vi "SEA-9811_ReceiverAndTransmitter_FPGA_9220_IO_simulated_NO_NIVS.vi"() -> ()   [LabVIEW 2015]
doc: "This example demonstrates the receiver's functionality. ARINC data can be received with up to 8 channels which can be configured regarding high- or low-speed data rate, label recognition, parity check, decoder functions or label bit order (CONFIG). Up to sixteen 8-bit labels can be stored for label recognition. Duplicate values if you need fewer labels. For more details, look at the RT frontend example.\n\nCopyright (c) 2013 S.E.A. Datentechnik GmbH, Germany"
uses:
  <vilib>/Platform/TimedLoop/XDataNode/timing_clust.ctl
  <vilib>/Platform/TimedLoop/XDataNode/nitl_modes.ctl
  <vilib>/Platform/TimedLoop/XDataNode/wakeup.ctl
  <vilib>/rvi/Emulation/niFpgaGetClockAttributes.vi
  <vilib>/rvi/Emulation/niFpgaSctlEmulationGetInTimedLoop.vi
  <vilib>/rvi/Emulation/niFpgaEmulationReportErrorSimple.vi
  <vilib>/rvi/Emulation/niFpgaCriticalErrorInLSC.vi
  <vilib>/rvi/Emulation/niFpgaProcessEmulError.vi
  GlobalVar.vi
  <vilib>/rvi/interface/RandomDataEmulation/niFpgaRandomDataHandleErrors.vi
  <vilib>/Platform/TimedLoop/XDataNode/XDataNode.xnode
  <vilib>/rvi/DataTransferAndStorage/Container/XNode/niFpgaContainer.xnode
  <vilib>/rvi/interface/RandomDataEmulation/nirviRandomDataFpgaReadWriteTemplate.vi
  <vilib>/rvi/eio/common/nirviEmuTemplateMethod_errors.vi
  <vilib>/eio/EIOPropertyNode/EIOPropertyNode.xnode
  <vilib>/eio/EIOMethodNode/EIOMethodNode.xnode
  <vilib>/eio/EIONode/EIONode.xnode
  <vilib>/rvi/eio/common/nirviEmuTemplatePropertyGet_errors.vi
  <vilib>/rvi/eio/common/nirviEmuTemplatePropertyGet_noerrors.vi
  <vilib>/rvi/eio/common/nirviEmuTemplatePropertySet_errors.vi
  <vilib>/rvi/eio/common/nirviEmuTemplatePropertySet_noerrors.vi
  <userlib>/FPGA Timekeeper 1.1b0/FPGA Timekeeper.lvlib
  <vilib>/Platform/TimedLoop/XDataNode/XDNodeRunTimeDep.lvlib
panel:
  in  "Rx Label Filter":u8[](array[numeric])=[0, 0, 0, 0, 0, 0, 0, 0, 0, 0, 0, 0, 0, 0, 0, 0]
  in  "RxSimRate(mSec)":u32=5 caption="Count(mSec)"
  out "Pulse":bool
  out "Counter":u32
  in  "AI0_threshold (V)":fxp<+/-,24,5>=5.0
  in  "Pulse length (ms)":u32
  in  "FPGA Loop rate (usec)":u16
  out "9220_AIs":fxp<+/-,24,5>[](array[numeric])
  out "Rx rate us":u32
  out "Elements in FIFO":u32
  out "FPGA Timekeeper time (ns)":u64
  out "FPGA Timekeeper locked":bool
  out "offset from RT time (ns)":i32
  in  "RT time (ns)":u64
  in  "Finished config":bool
  in  "Configure\nchannel":bool
  out "Rx Status":u16 format="%016b"
  out "Tx Status":u8 format="%08b"
  in  "Tx Data":u32=305419896 format="%08x"
  in  "Tx Config Data (TCR)":u16=8192 format="%04x"
  in  "Transmit Data":bool
  out "DMA Overflow":bool
  in  "Rx Channel Number":u8 max=7 step=1
  in  "Rx Config Data (RCR)":u16=32 format="%04x"
  # "Please refer to VI description for instructions!"
  # "Receiver Configuration"
  # "DMA Status"
  # "Transmitter"
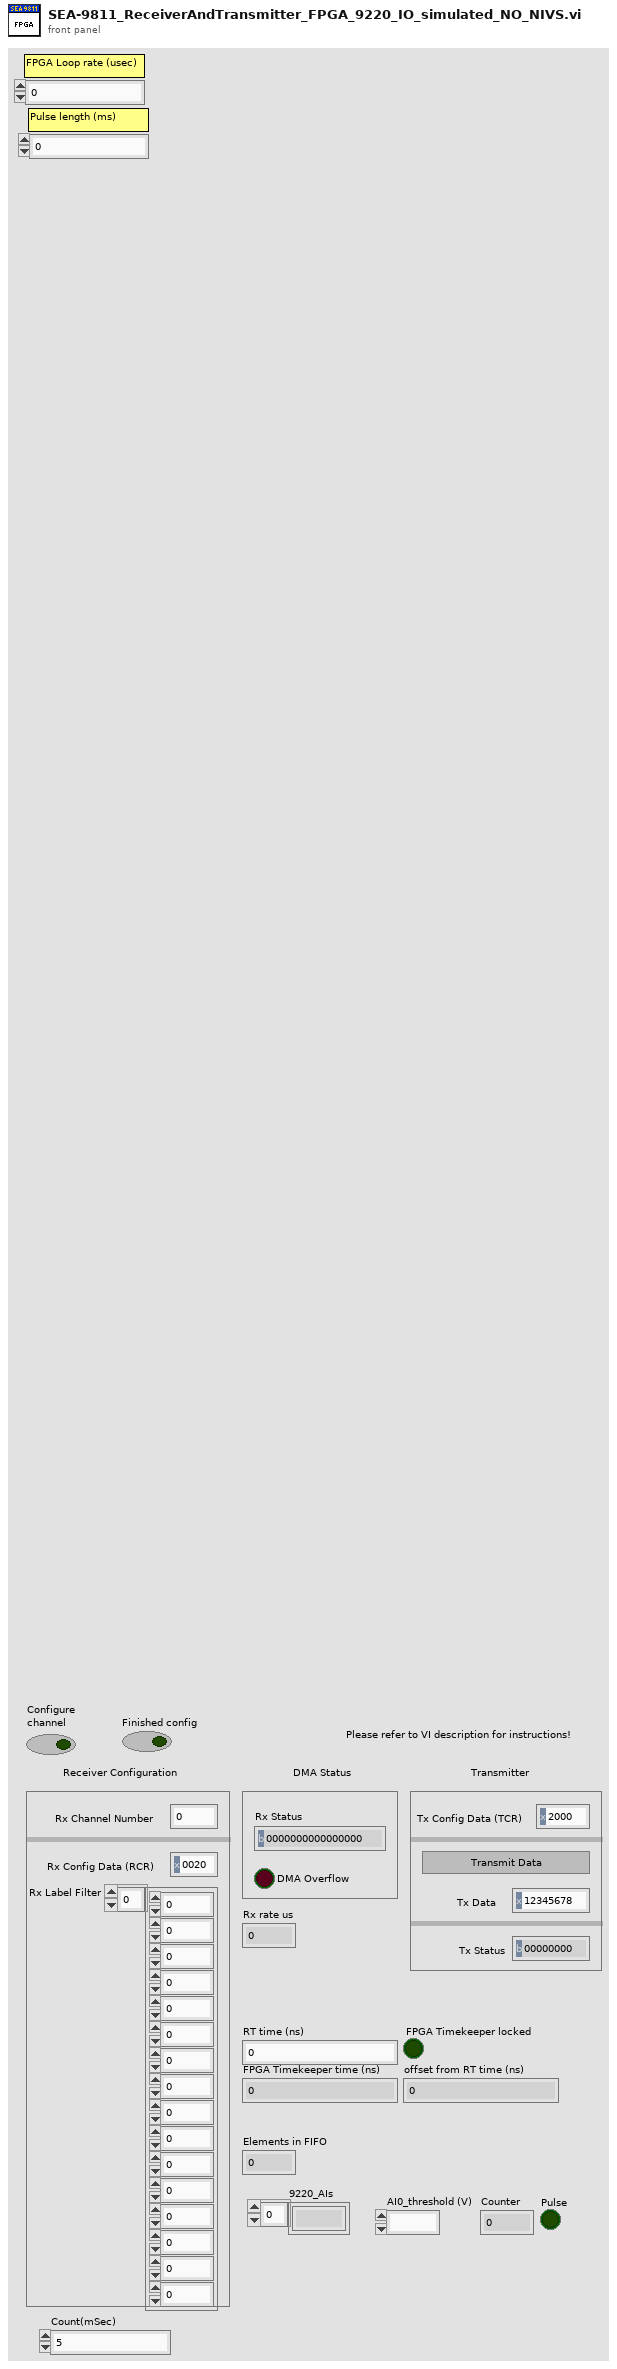
[diagram p1: front panel]
types:
  T1 = cluster{"Rx Label Filter[0]":u8, "Rx Label Filter[1]":u8, "Rx Label Filter[2]":u8, "Rx Label Filter[3]":u8, "Rx Label Filter[4]":u8, "Rx Label Filter[5]":u8, "Rx Label Filter[6]":u8, "Rx Label Filter[7]":u8, "Rx Label Filter[8]":u8, "Rx Label Filter[9]":u8, "Rx Label Filter[10]":u8, "Rx Label Filter[11]":u8, "Rx Label Filter[12]":u8, "Rx Label Filter[13]":u8, "Rx Label Filter[14]":u8, "Rx Label Filter[15]":u8}
  T2 = typedef "XDNodeRunTimeDep.lvlib/timing_clust.ctl" = cluster{"Expected End [f-1]":u64, "Actual End [f-1]":u64, "Finished Late? [f-1]":bool, "Expected End [i-1]":u64, "Actual End [i-1]":u64, "Finished Late? [i-1]":bool, "Expected Start [i]":u64, "Actual Start [i]":u64, "Expected Start [f]":u64, "Actual Start [f]":u64, "Source Name":string, "Structure Name":string, "Period":i64, "Deadline":i64, "Offset":i64, "Start":i64, "Priority":i32, "Timeout":i32, "Mode":T3, "Wakeup Reason":T4, "Error":errorcluster, "Source Type":string, "Secondary Source Type":string, "Global End Time":u64, "Global Start Time":u64, "Frame Duration":u64, "Iteration Duration":u64, "Assigned CPU":i32, "I/O Scan Engine Mode":u32}
  T3 = typedef "XDNodeRunTimeDep.lvlib/nitl_modes.ctl" = enum32{"No Change", "Process missed periods, maintain original phase", "Discard missed periods, maintain original phase", "Process missed periods, ignore original phase", "Discard missed periods, ignore original phase"}
  T4 = typedef "XDNodeRunTimeDep.lvlib/wakeup.ctl" = enum32{"Normal", "Aborted", "Asynchronous wakeup", "Timing source error", "Timed loop error", "Timeout"}
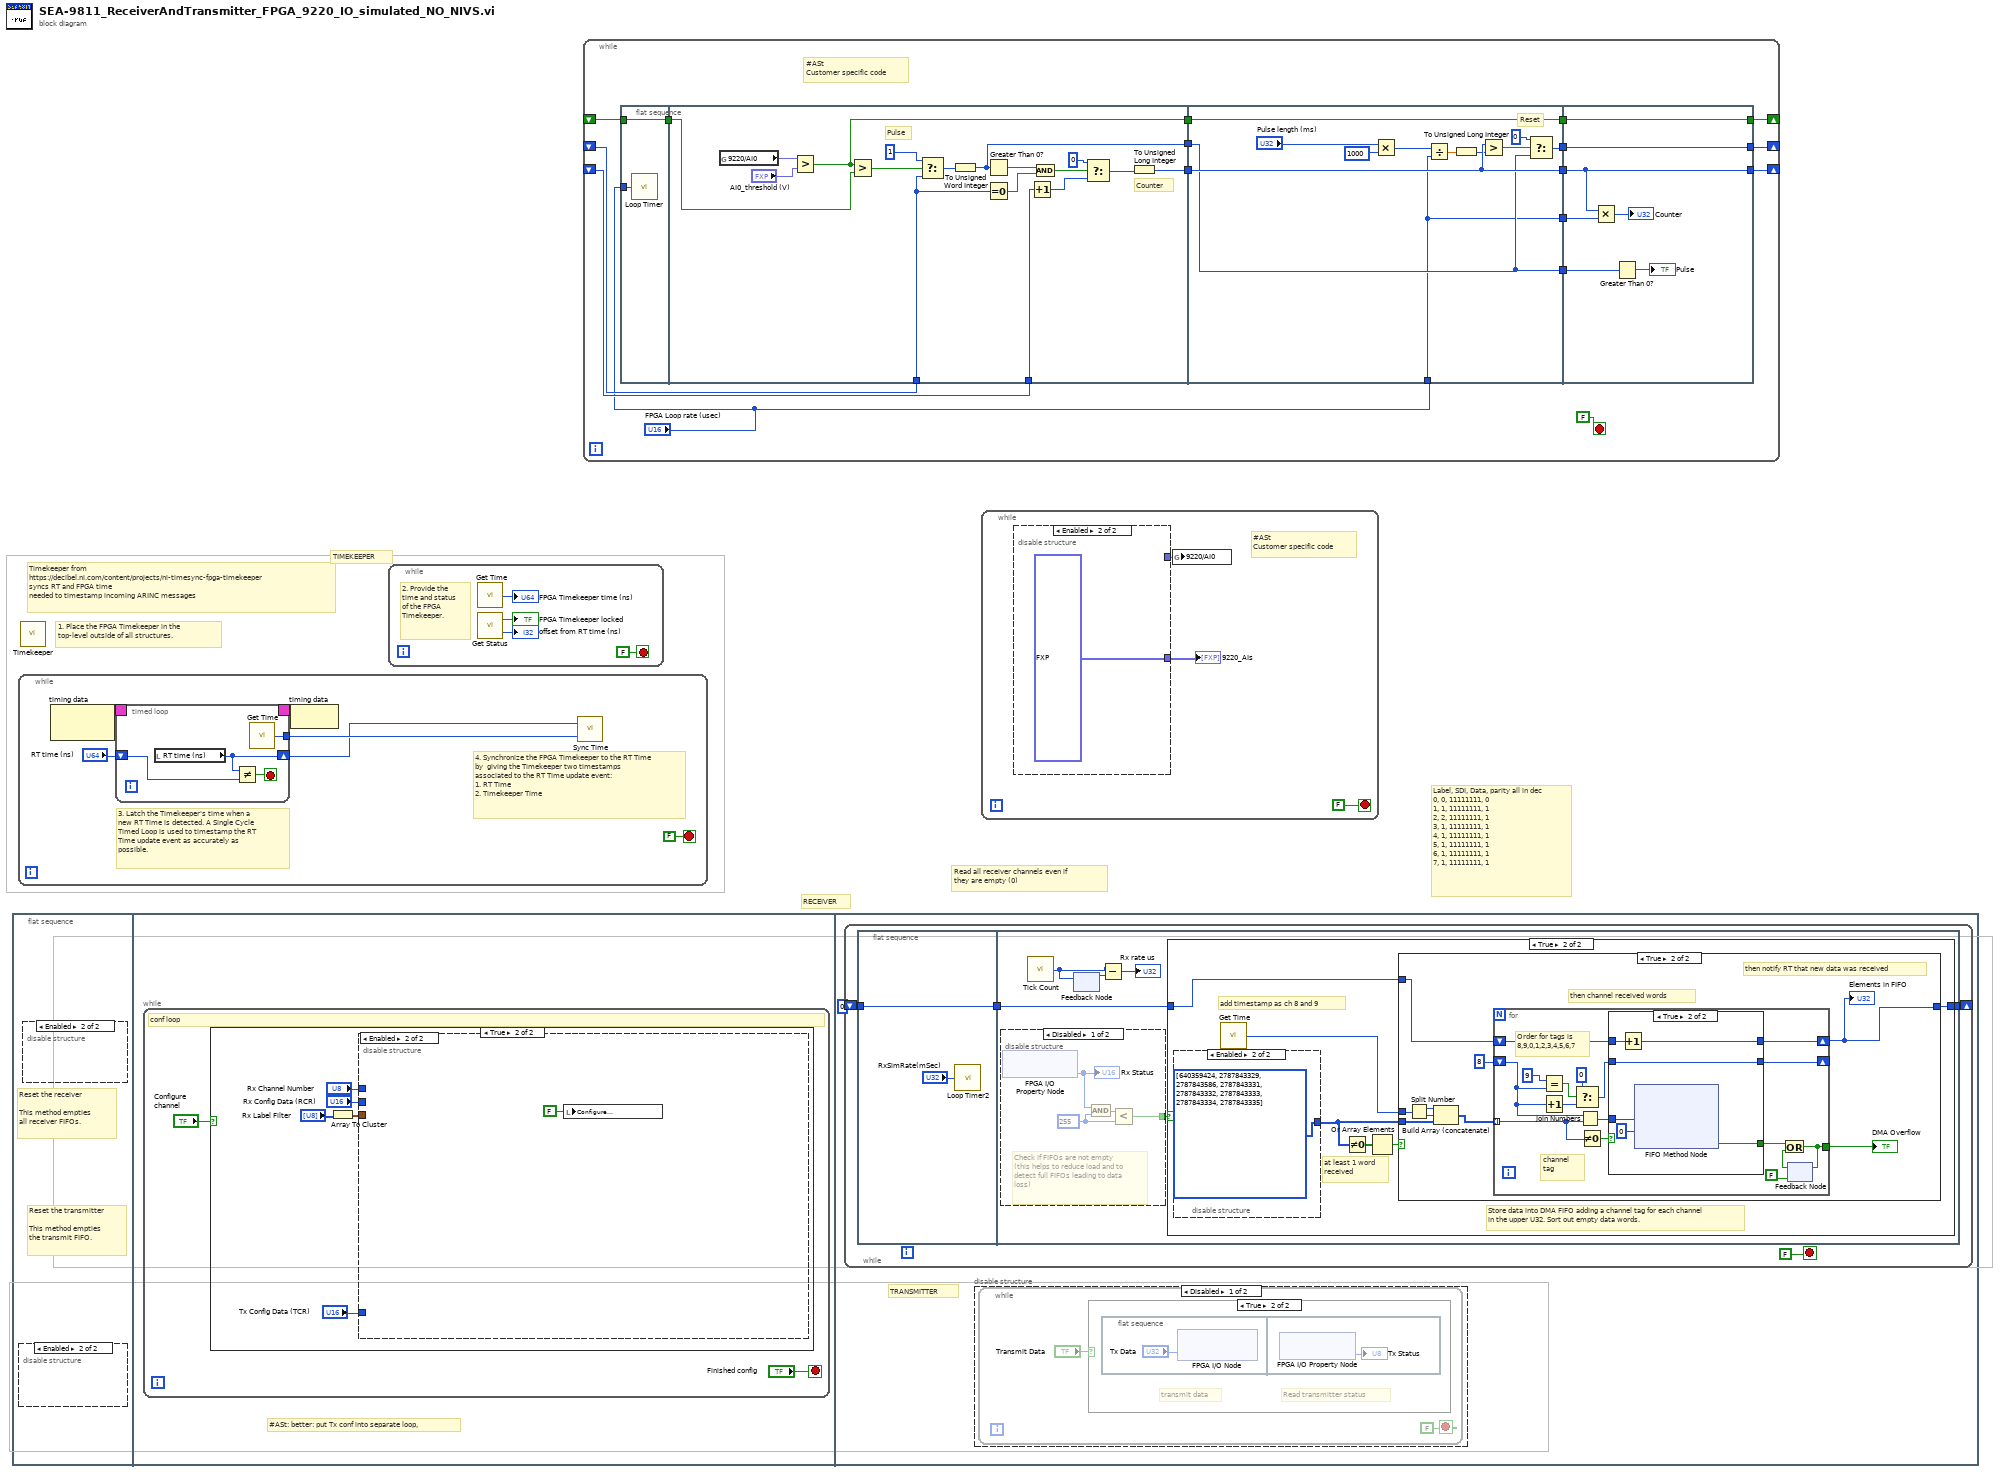
[diagram p0: block diagram]
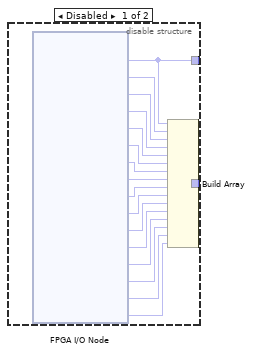
[diagram p2: hidden frame]
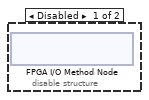
[diagram p3: hidden frame]
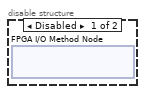
[diagram p4: hidden frame]
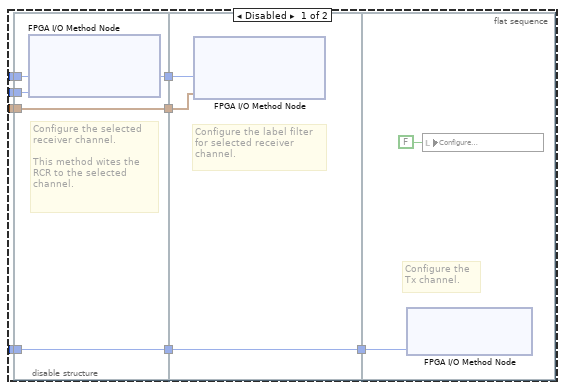
[diagram p6: hidden frame]
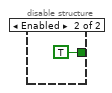
[diagram p9: hidden frame]
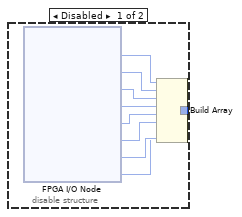
[diagram p11: hidden frame]
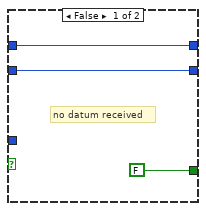
[diagram p13: hidden frame]
diagram:
  # "Label, SDI, Data, parity all in dec\n0, 0, 11111111, 0 \n1, 1, 11111111, 1 \n2, 2, 11111111, 1\n3, 1, 11111111, 1 \n4, 1, 11111111, 1 \n5, 1, 11111111, 1 \n6, 1, 11111111, 1 \n7, 1, 11111111, 1"
  # "Read all receiver channels even if they are empty (0)"
  # "TIMEKEEPER"
  # "Timekeeper from\nhttps://decibel.ni.com/content/projects/ni-timesync-fpga-timekeeper\nsyncs RT and FPGA time\nneeded to timestamp incoming ARINC messages"
  # "1. Place the FPGA Timekeeper in the top-level outside of all structures."
  # "RECEIVER"
  n1 = flat-sequence {
    frame #0 {
      # "Reset the transmitter\n\nThis method empties\nthe transmit FIFO."
      # "Reset the receiver\n\nThis method empties\nall receiver FIFOs."
      n2 = disable-structure shown="Enabled" {
        frame Disabled {
          n3 = xnode "FPGA I/O Method Node"() -> ()  [unwired: 1 in, 1 out]
        }
        frame Enabled {
        }
      }
      n4 = disable-structure shown="Enabled" {
        frame Disabled {
          n5 = xnode "FPGA I/O Method Node"() -> ()  [unwired: 1 in, 1 out]
        }
        frame Enabled {
        }
      }
    }
    frame #1 {
      # "#ASt: better: put Tx conf into separate loop,"
      n6 = while {
        stop <- "Finished config" stop-if-true
        # "conf loop"
        n7 = case shown="True" "Configure\nchannel" {
          frame False {
          }
          frame True {
            n8 = Array To Cluster(array="Rx Label Filter") -> (cluster=w3:T1)
            n9 = disable-structure shown="Enabled" {
              disable-tunnel: "Rx Channel Number" -> [w11 _]
              disable-tunnel: "Rx Config Data (RCR)" -> [w10 _]
              disable-tunnel: w3 -> [w9 _]
              disable-tunnel: "Tx Config Data (TCR)" -> [w8 _]
              frame Disabled {
                n10 = flat-sequence {
                  tunnel: w11 -> [w19]
                  tunnel: [w19] -> w15
                  tunnel: w10 -> [w18]
                  tunnel: [w17] -> w14
                  tunnel: w9 -> [w17]
                  tunnel: w8 -> [w16]
                  tunnel: [w16] -> w13
                  tunnel: w15 -> [w22]
                  tunnel: w14 -> [w21]
                  tunnel: [w20] -> w12
                  tunnel: w13 -> [w20]
                  tunnel: w12 -> [w24]
                  frame #0 {
                    # "Configure the selected\nreceiver channel.\n\nThis method wites the\nRCR to the selected\nchannel."
                    n11 = xnode "FPGA I/O Method Node"("Channel Number"=w19, "Control Register"=w18) -> ()  [unwired: 1 in, 1 out]
                  }
                  frame #1 {
                    # "Configure the label filter\nfor selected receiver\nchannel."
                    n12 = xnode "FPGA I/O Method Node"("Channel Number"=w22, "Label Filter"=w21) -> ()  [unwired: 1 in, 1 out]
                  }
                  frame #2 {
                    # "Configure the\nTx channel."
                    n13 = xnode "FPGA I/O Method Node"("Control Register"=w24) -> ()  [unwired: 1 in, 1 out]
                    n14 = local write "Configure\nchannel"(FALSE ("Configure\nchannel")) -> ()
                  }
                }
              }
              frame Enabled {
                n15 = local write "Configure\nchannel"(FALSE ("Configure\nchannel")) -> ()
              }
            }
          }
        }
      }
    }
    frame #2 {
      # "TRANSMITTER"
      n16 = while {
        shift-right: [w32] -> _
        shift-left: u32 0 -> [w33]
        stop <- FALSE stop-if-true
        n17 = flat-sequence {
          tunnel: w33 -> [w36]
          tunnel: [w36] -> w31
          tunnel: [w40] -> w32
          tunnel: w31 -> [w41]
          frame #0 {
            n18 = call "Loop Timer2"("Count(mSec)"="RxSimRate(mSec)") -> ()  [unwired: 1 out]
          }
          frame #1 {
            n19 = disable-structure shown="Disabled" {
              disable-tunnel: [w43 TRUE] -> w42
              frame Disabled {
                w44 = u16 255 ("y")
                # "Check if FIFOs are not empty\n(this helps to reduce load and to detect full FIFOs leading to data loss)"
                n20 = xnode "FPGA I/O Property Node"() -> ("Rx Status"=w46:u16)  [unwired: 1 in, 1 out]
                "Rx Status" <- w46
                n21 = And(x=w46, y=w44) -> (x .and. y?=w45:u16)
                n22 = Less?(x=w45, y=w44) -> (x < y?=w43:bool)
              }
              frame Enabled {
              }
            }
            n23 = call "Tick Count"() -> ("Tick Count(uSec)"=w37:u32)
            n24 = feedback #1() -> (w38:u32)  [unwired: 1 in]
            n25 = feedback-in #1(w37) -> ()
            n26 = Subtract(x=w37, y=w38) -> (x-y=→"Rx rate us":u32)
            n27 = case shown="True" w42 {
              tunnel: w41 -> [w48 w54]
              tunnel: [w48 w53] -> w40
              frame False {
              }
              frame True {
                # "add timestamp as ch 8 and 9"
                # "at least 1 word\nreceived"
                # "Store data into DMA FIFO adding a channel tag for each channel in the upper U32. Sort out empty data words."
                n28 = disable-structure shown="Enabled" {
                  disable-tunnel: [w55 u32[] [640359424, 2787843329, 2787843586, 2787843331, 2787843332, 2787843333, 2787843334, 2787843335]] -> w52
                  frame Disabled {
                    n29 = xnode "FPGA I/O Node"() -> ("Mod1/Rx0"=w57:u32, "Mod1/Rx1"=w58:u32, "Mod1/Rx2"=w59:u32, "Mod1/Rx3"=w60:u32, "Mod1/Rx4"=w61:u32, "Mod1/Rx5"=w62:u32, "Mod1/Rx6"=w63:u32, "Mod1/Rx7"=w56:u32)  [unwired: 8 in, 8 out]
                    n30 = Build Array(w57, w58, w59, w60, w61, w62, w63, w56) -> (w55:u32[])
                  }
                  frame Enabled {
                  }
                }
                n31 = call <userlib>:"Get Time.vi"() -> ("time (ns)"=w49:u64)
                n32 = Not Equal To 0?(x=w52) -> (x != 0?=w51:bool[])
                n33 = Or Array Elements(Boolean array=w51) -> (logical OR=w50:bool)
                n34 = case shown="True" w50 {
                  tunnel: w54 -> [w65 w66]
                  tunnel: [w65 w74] -> w53
                  tunnel: w52 -> [_ w71]
                  tunnel: w49 -> [_ w67]
                  frame False {
                  }
                  frame True {
                    # "then notify RT that new data was received"
                    # "then channel received words"
                    n35 = Split Number(x=w67) -> (hi(x)=w69:u32, lo(x)=w68:u32)
                    n36 = Build Array (concatenate)(w69, w68, w71) -> (w70:u32[])
                    n37 = for {
                      tunnel: w70 -> [w82] mode=indexing
                      tunnel: [w87] -> w73
                      shift-right: [w83] -> w74
                      shift-left: w66 -> [w84]
                      shift-right: [w75] -> _
                      shift-left: u32 8 ("hi") -> [w79]
                      # "Order for tags is\n8,9,0,1,2,3,4,5,6,7"
                      # "channel\ntag"
                      n38 = Equal?(x=u32 9, y=w79) -> (x = y?=w80:bool)
                      n39 = Increment(x=w79) -> (x+1=w81:u32)
                      n40 = Select(t=u32 0, s=w80, f=w81) -> (s? t:f=w76:u32)
                      n41 = Join Numbers(hi=w79, lo=w82) -> ((hi.lo)=w85:u64)
                      n42 = Not Equal To 0?(x=w82) -> (x != 0?=w86:bool)
                      n43 = case shown="True" w86 {
                        tunnel: [FALSE ("Timed Out?") w99] -> w88
                        tunnel: w85 -> [_ w96]
                        tunnel: w84 -> [w92 w98]
                        tunnel: [w92 w97] -> w83
                        tunnel: w76 -> [w91 w94]
                        tunnel: [w91 w94] -> w75
                        frame False {
                          # "no datum received"
                        }
                        frame True {
                          n44 = Increment(x=w98) -> (x+1=w97:u32)
                          n45 = xnode ("FIFO Method Node")("Element"=w96, "Timeout"=0) -> ("Timed Out?"=w99:bool)  [unwired: 1 in, 1 out]
                        }
                      }
                      n46 = feedback #2(FALSE) -> (w89:bool)
                      n47 = Or(x=w88, y=w89) -> (x .or. y?=w87:bool)
                      n48 = feedback-in #2(w87) -> ()
                    }
                    "DMA Overflow" <- w73
                    "Elements in FIFO" <- w74
                  }
                }
              }
            }
          }
        }
      }
      n49 = disable-structure shown="Disabled" {
        frame Disabled {
          n50 = while {
            stop <- FALSE stop-if-true
            n51 = case shown="True" "Transmit Data" {
              frame False {
              }
              frame True {
                # "Read transmitter status"
                # "transmit data"
                n52 = flat-sequence {
                  frame #0 {
                    n53 = xnode "FPGA I/O Node"("Mod1/Tx0"="Tx Data") -> ()  [unwired: 1 in, 1 out]
                  }
                  frame #1 {
                    n54 = xnode "FPGA I/O Property Node"() -> ("Tx Status"=→"Tx Status":u8)  [unwired: 1 in, 1 out]
                  }
                }
              }
            }
          }
        }
        frame Enabled {
        }
      }
    }
  }
  n55 = while {
    stop <- FALSE stop-if-true
    # "3. Latch the Timekeeper's time when a new RT Time is detected. A Single Cycle Timed Loop is used to timestamp the RT Time update event as accurately as possible."
    # "4. Synchronize the FPGA Timekeeper to the RT Time by  giving the Timekeeper two timestamps associated to the RT Time update event:\n1. RT Time\n2. Timekeeper Time"
    n56 = node-c288() -> (w105:T2)  [unwired: 1 in]
    n57 = timed-loop {
      timing: w105 -> [_]
      timing-out: [_] -> w104
      shift-right: [w106] -> w100
      shift-left: "RT time (ns)" -> [w107]
      tunnel: [w109] -> w103
      stop <- w108 stop-if-true
      n58 = local read "RT time (ns)"() -> (w106:u64)
      n59 = Not Equal?(x=w106, y=w107) -> (x != y?=w108:bool)
      n60 = call <userlib>:"Get Time.vi"() -> ("time (ns)"=w109:u64)
    }
    n61 = node-c288(w104) -> ()
    n62 = call <userlib>:"Sync Time.vi"("FPGA Timekeeper time (ns)"=w103, "time reference time (ns)"=w100) -> ()
  }
  n63 = call <userlib>:"Timekeeper.vi"() -> ()  [unwired: 12 in]
  n64 = while {
    stop <- FALSE stop-if-true
    # "2. Provide the time and status of the FPGA Timekeeper."
    n65 = call <userlib>:"Get Time.vi"() -> ("time (ns)"=→"FPGA Timekeeper time (ns)":u64)
    n66 = call <userlib>:"Get Status.vi"() -> ("FPGA Timekeeper locked"=→"FPGA Timekeeper locked":bool, "offset from time reference"=→"offset from RT time (ns)":i32)
  }
  n67 = while {
    shift-right: [w133] -> _
    shift-left: _ -> [w132]
    shift-right: [w131] -> _
    shift-left: _ -> [w126]
    shift-right: [w127] -> _
    shift-left: _ -> [w125]
    stop <- FALSE stop-if-true
    # "#ASt\nCustomer specific code"
    n68 = flat-sequence {
      tunnel: w132 -> [w136]
      tunnel: [w136] -> w124
      tunnel: "FPGA Loop rate (usec)" -> [w135]
      tunnel: [w137] -> w130
      tunnel: [w141] -> w129
      tunnel: [w140] -> w128
      tunnel: w126 -> [w144]
      tunnel: w125 -> [w143]
      tunnel: w124 -> [w153]
      tunnel: w128 -> [w161]
      tunnel: w129 -> [w155]
      tunnel: w130 -> [w165]
      tunnel: "FPGA Loop rate (usec)" -> [w154]
      tunnel: [w165] -> w122
      tunnel: [w164] -> w121
      tunnel: [w161] -> w120
      tunnel: [w155] -> w119
      tunnel: [w154] -> w118
      tunnel: [w169] -> w127
      tunnel: [w171] -> w131
      tunnel: [w172] -> w133
      tunnel: w122 -> [w172]
      tunnel: w121 -> [w171]
      tunnel: w120 -> [w169]
      tunnel: w119 -> [w170]
      tunnel: w118 -> [w168]
      frame #0 {
        n69 = call "Loop Timer"("Count(uSec)"=w135) -> ()  [unwired: 1 out]
      }
      frame #1 {
        # "Pulse"
        # "Counter"
        n70 = global read "GlobalVar.vi" "9220/AI0"() -> (w139:fxp<+/-,24,5>)
        n71 = Greater?(x=w139, y="AI0_threshold (V)") -> (0:w137:bool)
        n72 = Greater?(x=w137, y=w153) -> (0:w152:bool)
        n73 = Select(t=u8 1, s=w152, f=w144) -> (s? t:f=w150:u16)
        n74 = To Unsigned Word Integer(number=w150) -> (unsigned 16bit integer=w141:u16)
        n75 = Greater Than 0?(x=w141) -> (x > 0?=w149:bool)
        n76 = Equal To 0?(x=w144) -> (x = 0?=w148:bool)
        n77 = Increment(x=w143) -> (x+1=w145:u32)
        n78 = And(x=w149, y=w148) -> (x .and. y?=w147:bool)
        n79 = Select(t=u8 0, s=w147, f=w145) -> (s? t:f=w142:u32)
        n80 = To Unsigned Long Integer(number=w142) -> (unsigned 32bit integer=w140:u32)
      }
      frame #2 {
        # "Reset"
        n81 = Multiply(x="Pulse length (ms)", y=i16 1000) -> (x*y=w158:u32)
        n82 = Divide(x=w158, y=w154) -> (x/y=w156:sgl)
        n83 = To Unsigned Long Integer(number=w156) -> (unsigned 32bit integer=w157:u32)
        n84 = Greater?(x=w161, y=w157) -> (0:w162:bool)
        n85 = Select(t=u8 0, s=w162, f=w155) -> (s? t:f=w164:u16)
      }
      frame #3 {
        n86 = Multiply(x=w169, y=w168) -> (x*y=→"Counter":u32)
        n87 = Greater Than 0?(x=w170) -> (x > 0?=→"Pulse":bool)
      }
    }
  }
  n88 = while {
    stop <- FALSE stop-if-true
    # "#ASt\nCustomer specific code"
    n89 = disable-structure shown="Enabled" {
      disable-tunnel: [w177 fxp<+/-,24,5>[] [0.0, 1.0, 2.0, 0.0, 0.0, 0.0, 0.0, 0.0, 0.0, 0.0, 0.0, 0.0, 0.0, 0.0, 14.0, 15.0] ("9220_AIs")] -> w174
      disable-tunnel: [w176 _] -> w173
      frame Disabled {
        n90 = xnode "FPGA I/O Node"() -> ("9220/AI0"=w176:fxp<+/-,24,5>, "9220/AI1"=w192:fxp<+/-,24,5>, "9220/AI2"=w191:fxp<+/-,24,5>, "9220/AI3"=w190:fxp<+/-,24,5>, "9220/AI4"=w189:fxp<+/-,24,5>, "9220/AI5"=w188:fxp<+/-,24,5>, "9220/AI6"=w187:fxp<+/-,24,5>, "9220/AI7"=w186:fxp<+/-,24,5>, "9220/AI8"=w185:fxp<+/-,24,5>, "9220/AI9"=w184:fxp<+/-,24,5>, "9220/AI10"=w183:fxp<+/-,24,5>, "9220/AI11"=w182:fxp<+/-,24,5>, "9220/AI12"=w181:fxp<+/-,24,5>, "9220/AI13"=w180:fxp<+/-,24,5>, "9220/AI14"=w179:fxp<+/-,24,5>, "9220/AI15"=w178:fxp<+/-,24,5>)  [unwired: 16 in, 16 out]
        n91 = Build Array(w176, w192, w191, w190, w189, w188, w187, w186, w185, w184, w183, w182, w181, w180, w179, w178) -> (w177:fxp<+/-,24,5>[])
      }
      frame Enabled {
      }
    }
    "9220_AIs" <- w174
    n92 = global write "GlobalVar.vi" "9220/AI0"(w173) -> ()
  }
